vi "SVPO Peak Level (1 Ch DBL Array).vi"(6 "restart averaging? (F)":bool, 10 "sampling rate [Hz]":dbl=1.0, 11 "scaled signal [EU]":dbl[](array[numeric])) -> (1 "minimum level [EU]":dbl=nan, 2 "maximum level [EU]":dbl=nan, 3 "peak level [EU]":dbl=nan, 4 "duration [s]":dbl)   [LabVIEW 2017, in "SoundVib_VibrationLevel.lvlib"]
doc: "Uses a peak detector and computes the level of scaled time waveform signals and scaled array signals. <B>scaled signal [EU]</B> should have a zero DC component. You can attenuate the DC component with hardware AC-coupling filters and with software high-pass filters. Use this VI on embedded targets that have limited computational resources. Wire data to the scaled signal [EU] input to determine the polymorphic instance to use or manually select the instance."
uses:
  <vilib>/addons/Sound and Vibration/svt_Level/SoundVib_VibrationLevel.lvlib
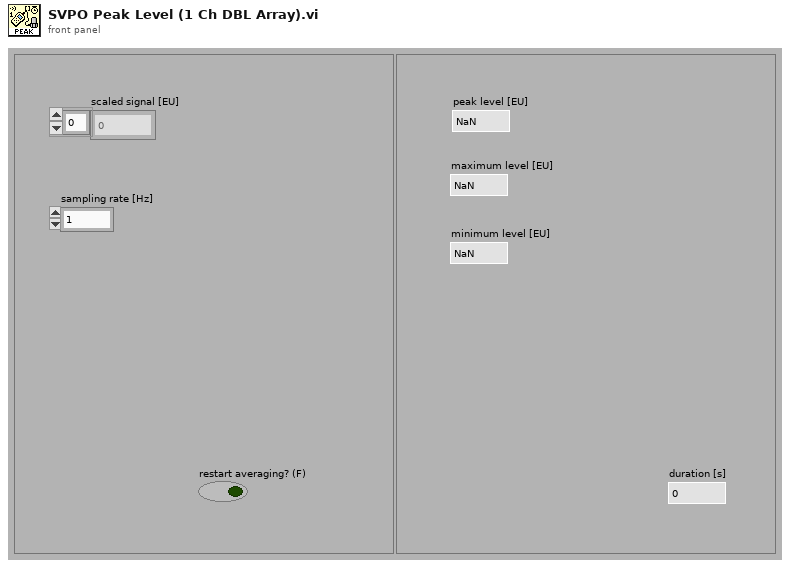
[diagram p1: front panel]
types:
  T1 = typedef "svc_Peak Level State.ctl" = cluster{"historical max":dbl, "historical min":dbl, "cumulative size":u64, "timestamp":timestamp}
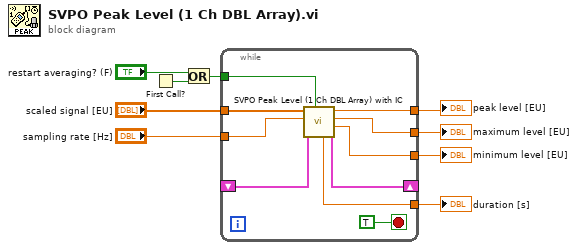
[diagram p0: block diagram]
diagram:
  n1 = First Call?() -> (First Call?: T/F=w6:bool)
  n2 = Or(x="restart averaging? (F)", y=w6) -> (x .or. y?=w4:bool)
  n3 = while {
    tunnel: "scaled signal [EU]" -> [w18]
    tunnel: [w16] -> w8
    tunnel: "sampling rate [Hz]" -> [w17]
    tunnel: w4 -> [w15]
    tunnel: [w14] -> w3
    tunnel: [w13] -> w2
    tunnel: [w12] -> w1
    shift-right: [w11] -> _
    shift-left: _ -> [w10]
    stop <- TRUE stop-if-true
    n4 = call <vilib>:"SVPO Peak Level (1 Ch DBL Array) with IC.vi"("restart averaging? (F)"=w15, "initial conditions"=w10, "sampling rate [Hz]"=w17, "scaled signal [EU]"=w18) -> ("final conditions"=w11:T1, "minimum level [EU]"=w12:dbl, "maximum level [EU]"=w13:dbl, "peak level [EU]"=w14:dbl, "duration [s]"=w16:dbl)  [unwired: 3 in]
  }
  "peak level [EU]" <- w3
  "duration [s]" <- w8
  "minimum level [EU]" <- w1
  "maximum level [EU]" <- w2
